vi "GetClassPath.vi"(8 "error in":errorcluster, 10 "class name":string, 11 "SystemConfigRepo in":refnum<class "SystemConfigRepo.lvclass">) -> (0 "error out":errorcluster, 2 "class path":path, 3 "SystemConfigRepo out":refnum<class "SystemConfigRepo.lvclass">)   [LabVIEW 2013, in "PL Framework Configuration Tool.lvlib" / "SystemConfigRepo.lvclass"]
doc: "Gets the path to the Class based on the Class Name. \nThe default behavior is build the path of the class on top of the class folder path. The name of the class and the folder it contains needs to be the same. A simple lookup from index and name would be the other option."
uses:
  SystemConfigRepo.lvclass
  Framework Configuration Classes/platypus configuration/class discovery singleton methods.ctl
  Framework Configuration Classes/platypus configuration/PLConfigurationSerializer.lvlib
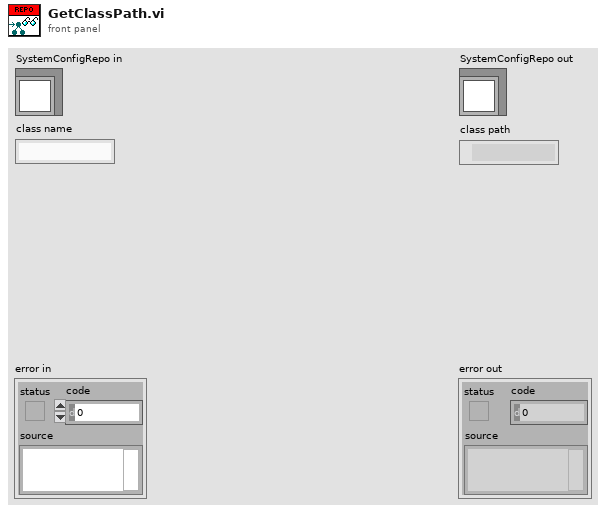
[diagram p1: front panel]
types:
  T1 = typedef "PLConfigurationSerializer.lvlib/class discovery singleton methods.ctl" = enum16{"add search paths", "load class by name", "list available classes", "get class path"}
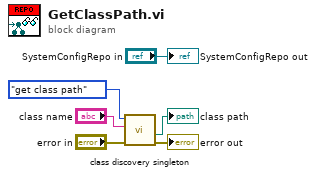
[diagram p0: block diagram]
diagram:
  n1 = call "class discovery singleton.vi"("error in"="error in", "Class Name"="class name", "method"=class_discovery_singleton_methods."get class path") -> ("error out"=→"error out":errorcluster, "class path"=→"class path":path)  [unwired: 5 in, 2 out]
  "SystemConfigRepo out" <- "SystemConfigRepo in"
